vi "Call Root.vi"(6 "Alias":string, 7 "Actor in":refnum<class "Actor.lvclass">, 10 "Root Actors":refnum<class "Root Actors.lvclass">) -> (0 "Error out":errorcluster, 2 "Actor out":refnum<class "Actor.lvclass">, 5 "Actor out":refnum<class "Actor.lvclass">)   [LabVIEW 2020, in "jettl.lvlib" / "Spawn.lvlib"]
uses:
  Spawn.lvlib
  Actor/Actor.lvclass
  Root Actors/Root Actors.lvclass
  Msg/Msg.lvclass
  Transport/Transport.lvclass
  Attributes Metadata/Attributes Metadata.lvclass
  Async Elements/Async Elements.lvclass
  Msgs.ctl
  jettl.lvlib
  Attributes.ctl
  Lifetime.ctl
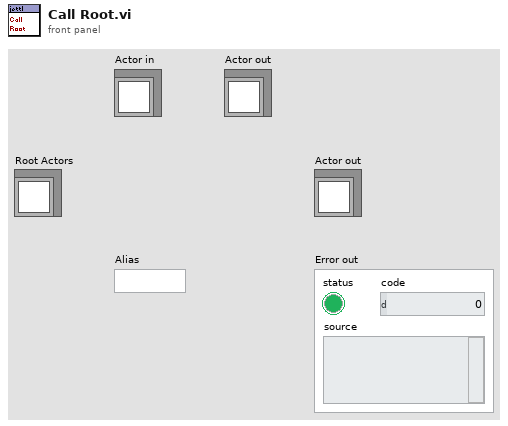
[diagram p1: front panel]
types:
  T1 = typedef "jettl.lvlib/Msgs.ctl" = set{refnum<class "Msg.lvclass">}
  T2 = typedef "jettl.lvlib/Attributes.ctl" = cluster{"Unified Msgs":T1, "Unified Leaf":bool, "Edge Actors":refnum<class "Actor.lvclass">[], "Core Actors":refnum<class "Actor.lvclass">[], "Root":bool, "Alias":string, "UID":i32, "Transport":refnum<class "Transport.lvclass">, "This VI":refnum<vi>, "Attributes Metadata":refnum<class "Attributes Metadata.lvclass">, "Post-Setup Actors":refnum<class "Actor.lvclass">[]}
  T3 = typedef "jettl.lvlib/Lifetime.ctl" = enum16{"Init", "Spawn", "Setup", "Teardown Before Running", "Running", "Stop Called", "Stopping With Children", "Stopping Without Children", "Teardown After Running", "Stopped"}
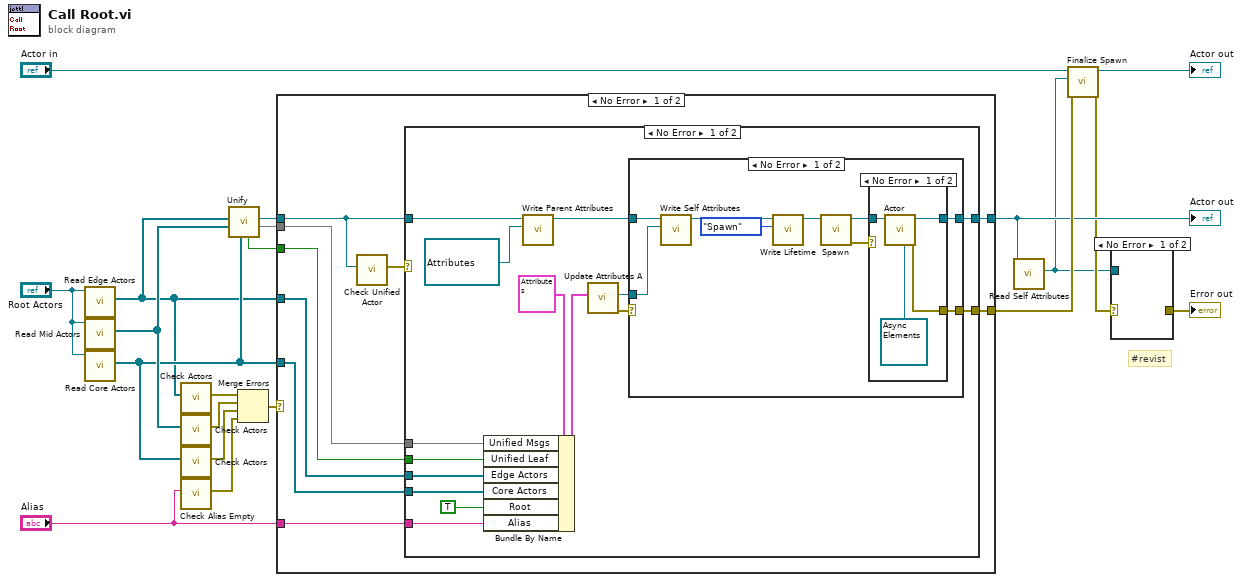
[diagram p0: block diagram]
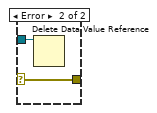
[diagram p6: hidden frame]
diagram:
  # "#revist"
  n1 = call-dynamic "Read Edge Actors.vi"("Root Actors in"="Root Actors") -> ("Edge Actors"=w1:refnum<class "Actor.lvclass">[])  [unwired: 10 in]
  n2 = call-dynamic "Read Mid Actors.vi"("Root Actors in"="Root Actors") -> ("Mid Actors"=w6:refnum<class "Actor.lvclass">[])  [unwired: 10 in]
  n3 = call-dynamic "Read Core Actors.vi"("Root Actors in"="Root Actors") -> ("Core Actors"=w5:refnum<class "Actor.lvclass">[])  [unwired: 10 in]
  n4 = call "Check Actors.vi"("Actors"=w1) -> ("Error"=w17:errorcluster)  [unwired: 10 in]
  n5 = call "Check Actors.vi"("Actors"=w6) -> ("Error"=w19:errorcluster)  [unwired: 10 in]
  n6 = call "Check Actors.vi"("Actors"=w5) -> ("Error"=w15:errorcluster)  [unwired: 10 in]
  n7 = call "Check Alias Empty.vi"("Alias"="Alias") -> ("Error"=w18:errorcluster)  [unwired: 10 in]
  n8 = call "Unify.vi"("Core Actors"=w5, "Mid Actors"=w6, "Edge Actors"=w1) -> ("Unified Msgs"=w3:T1, "Unified Actor"=w4:refnum<class "Actor.lvclass">, "Unified Leaf"=w2:bool)  [unwired: 6 in]
  n9 = Merge Errors(w17, w19, w15, w18) -> (w20:errorcluster)
  n10 = case shown="No Error" w20 {
    selector: w20 -> [_ w65]
    tunnel: [w27 w64] -> w10
    tunnel: [w28 w65] -> w13
    tunnel: w1 -> [w26 _]
    tunnel: "Alias" -> [w29 _]
    tunnel: w5 -> [w25 _]
    tunnel: w4 -> [w23 w64]
    tunnel: w3 -> [w22 _]
    tunnel: w2 -> [w21 _]
    frame No Error {
      n11 = call "Check Unified Actor.vi"("Unified Actor"=w23) -> ("Error"=w24:errorcluster)  [unwired: 10 in]
      n12 = case shown="No Error" w24 {
        selector: w24 -> [_ w63]
        tunnel: w29 -> [w43 _]
        tunnel: [w37 w63] -> w28
        tunnel: [w38 w62] -> w27
        tunnel: w26 -> [w41 _]
        tunnel: w25 -> [w40 _]
        tunnel: w23 -> [w34 w62]
        tunnel: w22 -> [w39 _]
        tunnel: w21 -> [w36 _]
        frame No Error {
          n13 = Bundle By Name(cluster=T2 {"Unified Msgs"={}, "Unified Leaf"=FALSE, "Edge Actors"=[], "Core Actors"=[], "Root"=FALSE, "Alias"="", "UID"=0, "Transport"=refnum, "This VI"=refnum, "Attributes Metadata"=refnum, "Post-Setup Actors"=[]} ("Attributes"), "Unified Msgs"=w39, "Unified Leaf"=w36, "Edge Actors"=w41, "Core Actors"=w40, "Root"=TRUE, "Alias"=w43) -> (w31:T2)
          n14 = call-dynamic "Write Parent Attributes.vi"("Parent Attributes"=refnum<data-value> refnum, "Actor in"=w34) -> ("Actor out"=w33:refnum<class "Actor.lvclass">)  [unwired: 9 in]
          n15 = call "Update Attributes A.vi"("Attributes"=w31) -> ("Error out"=w30:errorcluster, "Attributes out"=w35:refnum<data-value>)  [unwired: 9 in]
          n16 = case shown="No Error" w30 {
            selector: w30 -> [_ w61]
            tunnel: [w49 w60] -> w38
            tunnel: [w48 w61] -> w37
            tunnel: w35 -> [w46 _]
            tunnel: w33 -> [w45 w60]
            frame No Error {
              n17 = call-dynamic "Write Self Attributes.vi"("Self Attributes"=w46, "Actor in"=w45) -> ("Actor out"=w53:refnum<class "Actor.lvclass">)  [unwired: 9 in]
              n18 = call-dynamic "Write Lifetime.vi"("Lifetime"=Lifetime."Spawn", "Actor in"=w53) -> ("Actor out"=w52:refnum<class "Actor.lvclass">)  [unwired: 9 in]
              n19 = call-dynamic "Spawn.vi"("Actor in"=w52) -> ("Error out"=w47:errorcluster, "Actor out"=w50:refnum<class "Actor.lvclass">)  [unwired: 9 in]
              n20 = case shown="No Error" w47 {
                selector: w47 -> [_ w58]
                tunnel: w50 -> [w57 w59]
                tunnel: [w56 w59] -> w49
                tunnel: [w55 w58] -> w48
                frame No Error {
                  n21 = call-dynamic "Actor.vi"("Async Elements"=refnum<class "Async Elements.lvclass"> refnum, "Actor in"=w57) -> ("Error out"=w55:errorcluster, "Actor out"=w56:refnum<class "Actor.lvclass">)  [unwired: 8 in]
                }
                frame Error {
                }
              }
            }
            frame Error {
            }
          }
        }
        frame Error {
        }
      }
    }
    frame Error {
    }
  }
  "Actor out" <- w10
  n22 = call-dynamic "Read Self Attributes.vi"("Actor in"=w10) -> ("Self Attributes"=w7:refnum<data-value>)  [unwired: 10 in]
  n23 = call-dynamic "Finalize Spawn.vi"("Error in"=w13, "Attributes"=w7, "Actor in"="Actor in") -> ("Error out"=w9:errorcluster, "Actor out"=→"Actor out":refnum<class "Actor.lvclass">)  [unwired: 7 in]
  n24 = case shown="No Error" w9 {
    selector: w9 -> [_ w67]
    tunnel: [_ w67] -> w8
    tunnel: w7 -> [_ w66]
    frame No Error {
    }
    frame Error {
      n25 = Delete Data Value Reference(data value reference=w66) -> ()  [unwired: 1 in, 2 out]
    }
  }
  "Error out" <- w8
